vi "Block Write Iterator.vi"(8 "error in (no error)":errorcluster, 9 "Iterations (1000)":i32=110, 10 "Channel Count":i32, 11 "GE 5565PIORC in":refnum<class "GE 5565PIORC.lvclass">) -> (0 "error out":errorcluster, 1 "Histogram Graph":T1(graph), 2 "Metrics":T2 {"Transfer Rate" format="%.2pB/s"; "Duration Std. Dev." format="%.0f µs"; "Duration Average" format="%.0f µs"}, 3 "GE 5565PIORC out":refnum<class "GE 5565PIORC.lvclass">)   [LabVIEW 2016]
uses:
  Source/GE 5565PIORC/GE 5565PIORC.lvclass
  Controls/Throughput Metrics.ctl
  Source/GE 5565PIORC/GE 5565PIORC.lvclass/GE 5565PIORC.ctl
  Source/GE 5565PIORC/VIs/Binary Operations/Align to 8-byte Boundary.vi
  Source/GE 5565PIORC/VIs/Binary Operations/Align to 16-byte Boundary.vi
  Source/GE 5565PIORC/VIs/DMA/DMA.Transfer Size.vi
  Source/GE 5565PIORC/VIs/Registers/Local Configuration.PCI Address.Set.vi
  Source/GE 5565PIORC/VIs/Registers/Local Configuration.DMADPR0.First Descriptor Address.Set.vi
  Source/GE 5565PIORC/VIs/DMA/DMA.Scatter-Gather.Link Block Descriptors.vi
  Source/GE 5565PIORC/VIs/DMA/DMA.Scatter-Gather.Commit Blocks.vi
  Source/GE 5565PIORC/VIs/Registers/Local Configuration.Local Address.Set.vi
  Source/GE 5565PIORC/VIs/Registers/Local Configuration.Transfer Size.Set.vi
  Source/GE 5565PIORC/VIs/Registers/Local Configuration.DMADPR0.Transfer Direction.Set.vi
  Source/GE 5565PIORC/VIs/Registers/Local Configuration.DMAMODE0.Scatter-Gather Enable.Set.vi
  <vilib>/Utility/error.llb/Clear Errors.vi
  Source/GE 5565PIORC/VIs/Registers/Local Configuration.DMACSR0.DMA Start.Set.vi
  Source/GE 5565PIORC/VIs/Interrupts/Wait for PXI Interrupt Events.vi
  Source/GE 5565PIORC/VIs/Registers/Local Configuration.DMACSR0.DMA Clear Interrupt.Set.vi
  Source/GE 5565PIORC/VIs/Registers/Local Configuration.Get Register Offset.vi
  Source/GE 5565PIORC/VIs/Binary Operations/Set Bits.vi
  Source/GE 5565PIORC/VIs/Binary Operations/Set Bits U32.vi
  Source/GE 5565PIORC/VIs/Binary Operations/Get Bits.vi
  Source/GE 5565PIORC/VIs/Binary Operations/Get Bits U32.vi
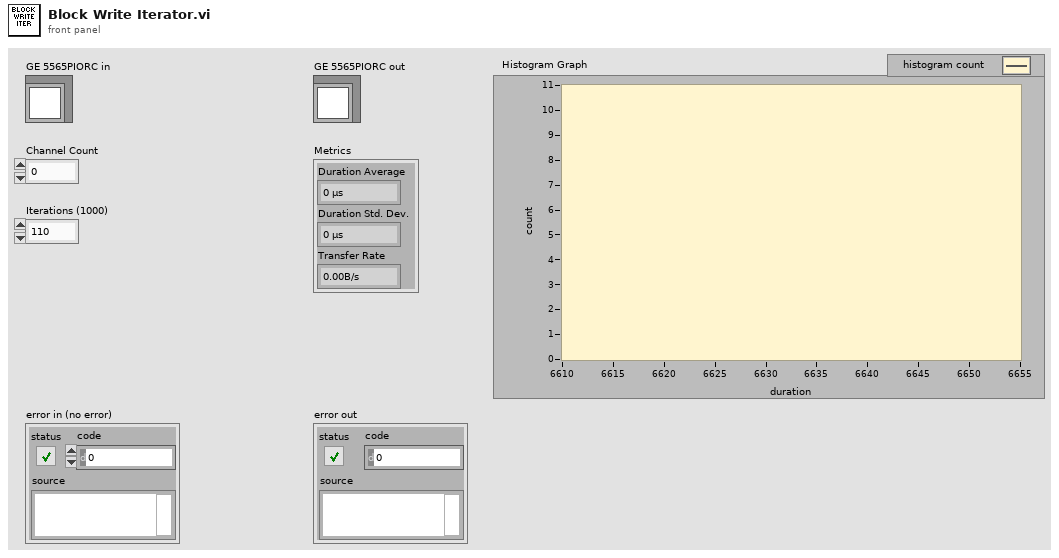
[diagram p1: front panel]
types:
  T1 = cluster{"X Values":dbl[], "Histogram: h(x)":i32[]}
  T2 = typedef "Throughput Metrics.ctl" = cluster{"Duration Average":u32, "Duration Std. Dev.":u32, "Transfer Rate":dbl}
  T3 = typedef "GE 5565PIORC.lvclass/DMA Block Descriptor.ctl" = cluster{"descriptor ptr (VISA)":u32, "descriptor size":u32, "descriptor ptr (aligned)":u32, "data ptr (lower)":u32, "data ptr (upper)":u32, "data size":u32, "next descriptor ptr":u32}
  T4 = typedef "GE 5565PIORC.lvclass/DMA Transfer Spec.ctl" = cluster{"RFM Address":u32, "Block Descriptors":T3[]}
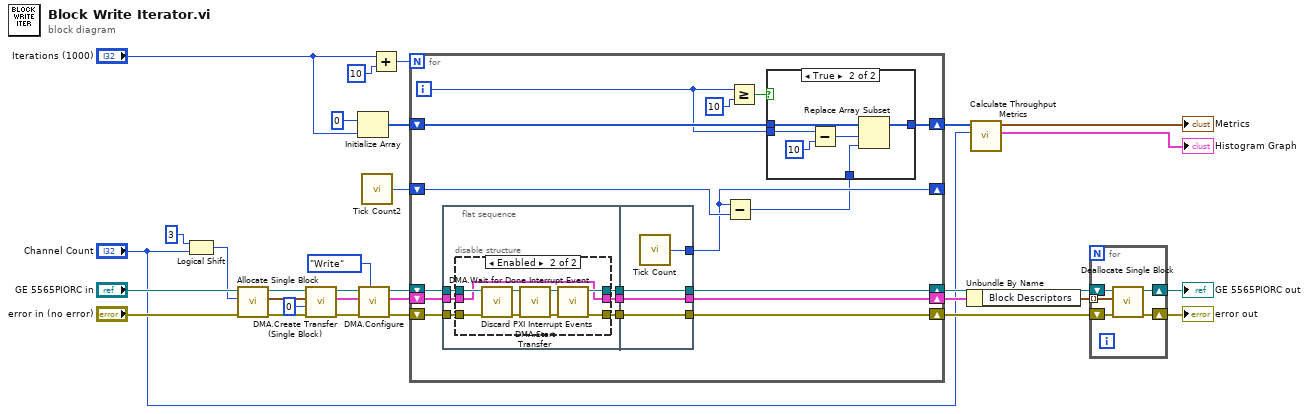
[diagram p0: block diagram]
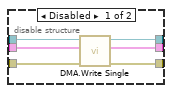
[diagram p2: hidden frame]
diagram:
  n1 = Logical Shift(y=i16 3, x="Channel Count") -> (x << y=w18:i32)
  n2 = call "Allocate Single Block.vi"("error in (no error)"="error in (no error)", "size (bytes)"=w18, "GE 5565PIORC in"="GE 5565PIORC in") -> ("error out"=w20:errorcluster, "Block Descriptor"=w17:T3, "GE 5565PIORC out"=w19:refnum<class "GE 5565PIORC.lvclass">)  [unwired: 6 in]
  n3 = call "DMA.Create Transfer (Single Block).vi"("error in (no error)"=w20, "RFM Offset"=u32 0, "Block Descriptor"=w17, "GE 5565PIORC in"=w19) -> ("error out"=w5:errorcluster, "DMA Transfer Spec"=w4:T4, "GE 5565PIORC out"=w3:refnum<class "GE 5565PIORC.lvclass">)  [unwired: 4 in, 1 out]
  n4 = Initialize Array(u32 0 ("x-y"), "Iterations (1000)") -> (w14:u32[])
  n5 = call "DMA.Configure.vi"("Transfer Direction"=enum16{"Write", "Read"}."Write", "error in (no error)"=w5, "DMA Transfer Spec"=w4, "GE 5565PIORC"=w3) -> ("error out"=w7:errorcluster, "DMA Transfer Spec out"=w6:T4, "GE 5565PIORC out"=w2:refnum<class "GE 5565PIORC.lvclass">)  [unwired: 5 in]
  n6 = call "Tick Count2"() -> ("Tick Count(uSec)"=w24:u32)
  n7 = Add(x="Iterations (1000)", y=10) -> (x+y=w31:i32)
  n8 = for {
    N: w31 -> [_]
    shift-right: [w42] -> _
    shift-left: w24 -> [w43]
    shift-right: [w45] -> w25
    shift-left: w2 -> [w48]
    shift-right: [w44] -> w26
    shift-left: w7 -> [w47]
    shift-right: [w40] -> w11
    shift-left: w14 -> [w41]
    shift-right: [w38] -> w13
    shift-left: w6 -> [w46]
    i -> [w39]
    n9 = flat-sequence {
      tunnel: w48 -> [w54]
      tunnel: w47 -> [w53]
      tunnel: w46 -> [w52]
      tunnel: [w49] -> w37
      tunnel: [w50] -> w36
      tunnel: [w51] -> w35
      tunnel: [w73] -> w45
      tunnel: w37 -> [w72]
      tunnel: [w72] -> w44
      tunnel: [w71] -> w42
      tunnel: w36 -> [w70]
      tunnel: [w70] -> w38
      tunnel: w35 -> [w73]
      frame #0 {
        n10 = disable-structure shown="Enabled" {
          disable-tunnel: w54 -> [w60 w65]
          disable-tunnel: w53 -> [w59 w64]
          disable-tunnel: w52 -> [w58 w61]
          disable-tunnel: [w57 w63] -> w51
          disable-tunnel: [w56 w61] -> w50
          disable-tunnel: [w55 w62] -> w49
          frame Disabled {
            n11 = call "DMA.Write Single.vi"("error in (no error)"=w59, "DMA Transfer Spec"=w58, "GE 5565PIORC"=w60) -> ("error out"=w55:errorcluster, "DMA Transfer Spec out"=w56:T4, "GE 5565PIORC out"=w57:refnum<class "GE 5565PIORC.lvclass">)  [unwired: 5 in, 1 out]
          }
          frame Enabled {
            n12 = call "Discard PXI Interrupt Events.vi"("error in (no error)"=w64, "GE 5565PIORC in"=w65) -> ("error out"=w68:errorcluster, "GE 5565PIORC out"=w67:refnum<class "GE 5565PIORC.lvclass">)  [unwired: 8 in]
            n13 = call "DMA.Start Transfer.vi"("error in (no error)"=w68, "GE 5565PIORC"=w67) -> ("error out"=w69:errorcluster, "GE 5565PIORC out"=w66:refnum<class "GE 5565PIORC.lvclass">)  [unwired: 8 in]
            n14 = call "DMA.Wait for Done Interrupt Event.vi"("error in (no error)"=w69, "GE 5565PIORC"=w66) -> ("error out"=w62:errorcluster, "GE 5565PIORC out"=w63:refnum<class "GE 5565PIORC.lvclass">)  [unwired: 7 in, 1 out]
          }
        }
      }
      frame #1 {
        n15 = call "Tick Count"() -> ("Tick Count(uSec)"=w71:u32)
      }
    }
    n16 = Subtract(x=w42, y=w43) -> (x-y=w32:u32)
    n17 = Greater Or Equal?(x=w39, y=10) -> (x >= y?=w33:bool)
    n18 = case shown="True" w33 {
      tunnel: w41 -> [w74 w80]
      tunnel: [w74 w79] -> w40
      tunnel: w39 -> [_ w78]
      tunnel: w32 -> [_ w75]
      frame False {
      }
      frame True {
        n19 = Subtract(x=w78, y=10) -> (x-y=w76:i32)
        n20 = Replace Array Subset(array=w80, new element=w75, index=w76) -> (w79:u32[])
      }
    }
  }
  n21 = Unbundle By Name(w13) -> ("Block Descriptors"=w12:T3[])
  n22 = call "Calculate Throughput Metrics.vi"("Channel Count"="Channel Count", "Durations"=w11) -> ("Histogram Graph"=→"Histogram Graph":T1, "Metrics"=→"Metrics":T2)  [unwired: 8 in]
  n23 = for {
    tunnel: w12 -> [w81] mode=indexing
    shift-right: [w85] -> w28
    shift-left: w26 -> [w83]
    shift-right: [w84] -> w27
    shift-left: w25 -> [w82]
    n24 = call "Deallocate Single Block.vi"("error in (no error)"=w83, "Block Descriptor"=w81, "GE 5565PIORC in"=w82) -> ("error out"=w85:errorcluster, "GE 5565PIORC out"=w84:refnum<class "GE 5565PIORC.lvclass">)  [unwired: 7 in]
  }
  "error out" <- w28
  "GE 5565PIORC out" <- w27
